vi "Moisture_Update.vi"(0 "task/channels in":refnum<k21>, 5 "Offset (V)":dbl format="%0.2p", 7 "Dither (V)":dbl format="%0.2p", 11 "Error In":errorcluster) -> (4 "task out":refnum<k21>, 15 "Error Out":errorcluster)   [LabVIEW 2014]
uses:
  <vilib>/DAQmx/write.llb/DAQmx Write (Analog Wfm 1Chan NSamp).vi
  <vilib>/measure/NI_MABase.lvlib
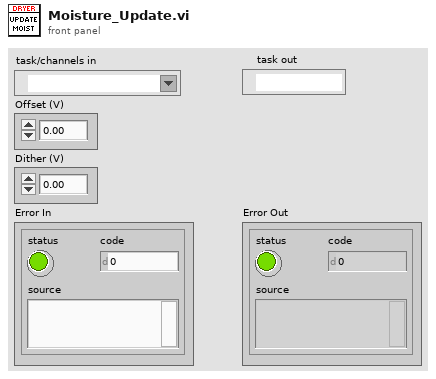
[diagram p1: front panel]
types:
  T1 = enum16{"Sine Wave", "Triangle Wave", "Square Wave", "Sawtooth Wave"}
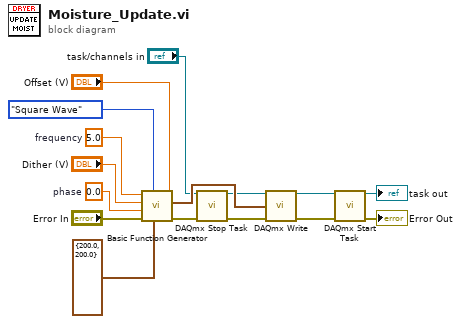
[diagram p0: block diagram]
diagram:
  w11 = 5.0  # frequency
  w12 = 0.0  # phase
  n1 = call <vilib>:"Basic Function Generator.vi"("offset"="Offset (V)", "sampling info"=cluster{"Fs":dbl, "#s":dbl} {"Fs"=200.0, "#s"=200.0} ("output cluster"), "signal type"=T1."Square Wave", "error in (no error)"="Error In", "phase"=w12, "amplitude"="Dither (V)", "frequency"=w11) -> ("error out"=w2:errorcluster, "signal out"=w15:waveform(dbl))  [unwired: 2 in, 1 out]
  n2 = call <vilib>:"DAQmx Stop Task.vi"("task/channels in"="task/channels in", "error in"=w2) -> ("task out"=w4:refnum<k21>, "error out"=w3:errorcluster)  [unwired: 12 in]
  n3 = call-poly <vilib>:"DAQmx Write.vi"("task/channels in"=w4, "data"=w15, "error in"=w3) -> ("task out"=w9:refnum<k21>, "error out"=w8:errorcluster)  [unwired: 10 in, 1 out]
  n4 = call <vilib>:"DAQmx Start Task.vi"("task/channels in"=w9, "error in"=w8) -> ("task out"=→"task out":refnum<k21>, "error out"=→"Error Out":errorcluster)  [unwired: 12 in]
